vi "IRAdressData.vi"() -> ()   [LabVIEW 2026]
panel:
  out "NICHT x?":u8 format="%x"
  out "Data":bool[](array[boolean])
  in  "Data":u8 format="%x"
  out "Adresse":bool[](array[boolean])
  in  "Adresse":u8 format="%x"
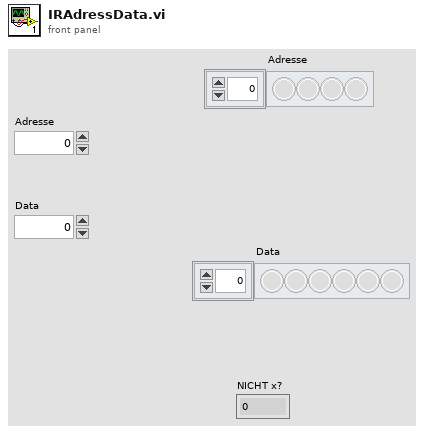
[diagram p1: front panel]
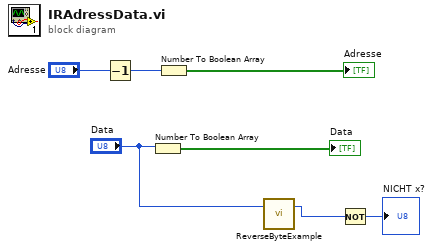
[diagram p0: block diagram]
diagram:
  n1 = Decrement(x="Adresse") -> (x-1=w4:u8)
  n2 = Number To Boolean Array(number="Data") -> (Boolean array=→"Data":bool[])
  n3 = Number To Boolean Array(number=w4) -> (Boolean array=→"Adresse":bool[])
  n4 = call "ReverseByteExample.vi"("Numeric"="Data") -> ("Numeric 2"=w2:u8)  [unwired: 2 in]
  n5 = Not(x=w2) -> (.not. x?=→"NICHT x?":u8)
